vi "fgt get sensor Bypass Valve.vi"(8 "error in (no error)":errorcluster, 11 "sensorIndex":u32) -> (0 "error out":errorcluster, 3 "open?":bool)   [LabVIEW 2016, in "fgt_SDK.lvlib"]
doc: "Returns the current state of the bypass valve. This feature is only available on NIFS devices."
uses:
  fgt_SDK.lvlib
  dlls/fgt_SDK_32.dll
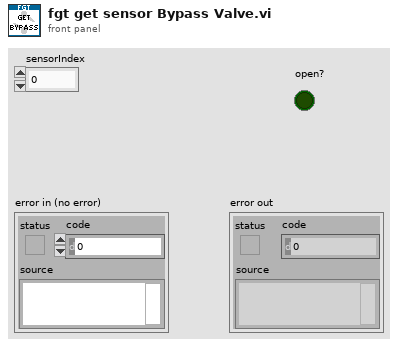
[diagram p1: front panel]
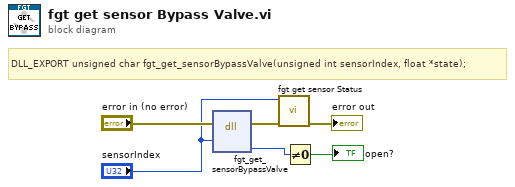
[diagram p0: block diagram]
diagram:
  # "DLL_EXPORT unsigned char fgt_get_sensorBypassValve(unsigned int sensorIndex, float *state);"
  n1 = dll-call lib="C:/projects/SDK/fgt-sdk-labview/dlls/fgt_SDK_*.*" fn="fgt_get_sensorBypassValve"(error in="error in (no error)", "sensorIndex"="sensorIndex") -> (error out=w5:errorcluster, "value"=w2:u8)  [unwired: 5 in, 1 out]
  n2 = call "fgt get sensor Status.vi"("error in (no error)"=w5, "pressureIndex"="sensorIndex") -> ("error out"=→"error out":errorcluster)  [unwired: 9 in]
  n3 = Not Equal To 0?(x=w2) -> (x != 0?=→"open?":bool)
